vi "Reveal World.vi"(6 "radius":i32 min=0, 8 "y":i32 min=0, 9 "x":i32 min=0, 10 "cost in":dbl[][](array[numeric]), 11 "map reference in":refnum<data-value>) -> (2 "cost out":dbl[][](array[numeric]), 3 "map reference in 2":refnum<data-value>)   [LabVIEW 2012]
uses:
  <vilib>/robotics/Navigation/shared/WorldMap/OccupancyGridWorldMap/NI_Robotics_OccupancyGridWorldMap.lvclass
panel:
  in  "error in (no error)":errorcluster
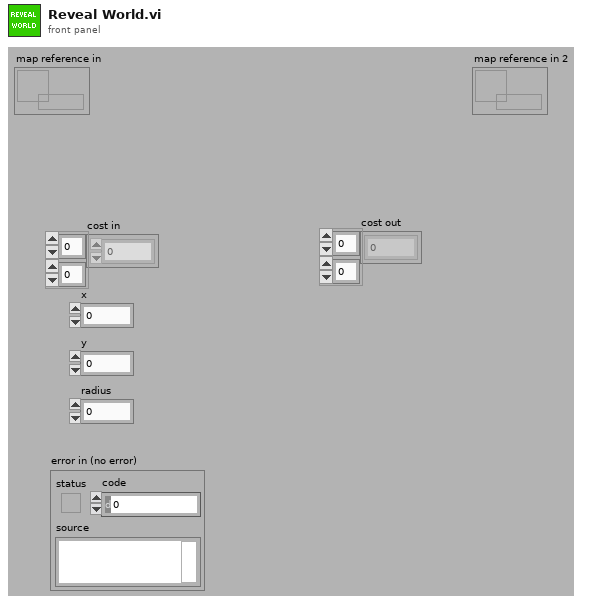
[diagram p1: front panel]
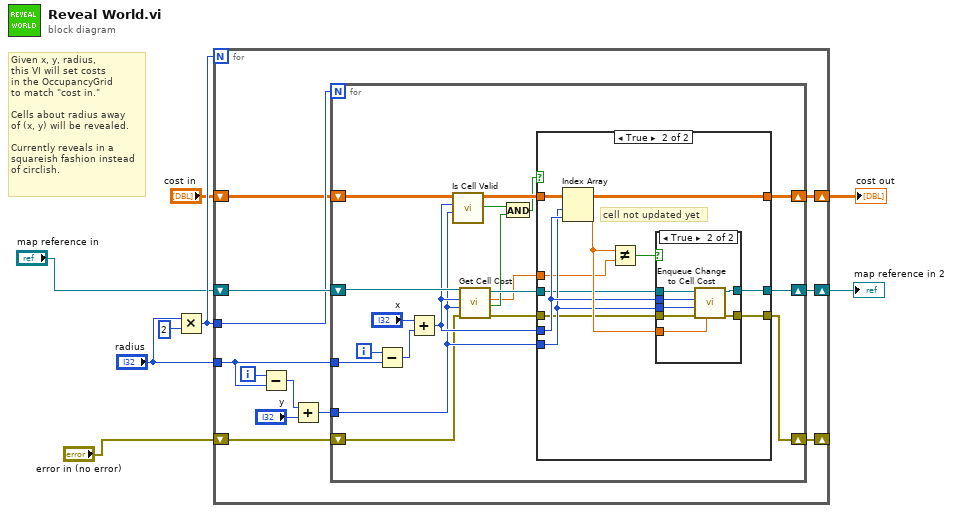
[diagram p0: block diagram]
diagram:
  # "Given x, y, radius,\nthis VI will set costs\nin the OccupancyGrid\nto match \"cost in.\"\n\nCells about radius away\nof (x, y) will be revealed.\n\nCurrently reveals in a \nsquareish fashion instead\nof circlish."
  n1 = Multiply(x="radius", y=2) -> (x*y=w6:i32)
  n2 = for {
    N: w6 -> [_]
    shift-right: [w19] -> w2
    shift-left: "map reference in" -> [w20]
    tunnel: w6 -> [w18]
    tunnel: "radius" -> [w16]
    shift-right: [w14] -> w4
    shift-left: "cost in" -> [w15]
    shift-right: [w9] -> _
    shift-left: "error in (no error)" -> [w10]
    i -> [w17]
    n3 = Subtract(x=w17, y=w16) -> (x-y=w13:i32)
    n4 = Add(x=w13, y="y") -> (x+y=w11:i32)
    n5 = for {
      N: w18 -> [_]
      shift-right: [w39] -> w19
      shift-left: w20 -> [w29]
      tunnel: w16 -> [w37]
      tunnel: w11 -> [w26]
      shift-right: [w34] -> w14
      shift-left: w15 -> [w36]
      shift-right: [w21] -> w9
      shift-left: w10 -> [w23]
      i -> [w38]
      n6 = Subtract(x=w38, y=w37) -> (x-y=w32:i32)
      n7 = Add(x="x", y=w32) -> (x+y=w27:i32)
      n8 = call "Is Cell Valid.vi"("y"=w26, "x"=w27, "cost in"=w36) -> ("Valid"=w30:bool, "cost out"=w35:dbl[][])  [unwired: 7 in]
      n9 = call <vilib>:"Get Cell Cost.vi"("error in (no error)"=w23, "y"=w26, "x"=w27, "map reference in"=w29) -> ("error out"=w22:errorcluster, "found?"=w25:bool, "cost"=w24:dbl, "map reference out"=w28:refnum<data-value>)  [unwired: 4 in]
      n10 = And(x=w30, y=w25) -> (x .and. y?=w33:bool)
      n11 = case shown="True" w33 {
        tunnel: [w42 w52] -> w39
        tunnel: w28 -> [w42 w46]
        tunnel: w27 -> [_ w49]
        tunnel: w26 -> [_ w48]
        tunnel: w35 -> [w41 w43]
        tunnel: [w41 w43] -> w34
        tunnel: w24 -> [_ w47]
        tunnel: w22 -> [w40 w45]
        tunnel: [w40 w44] -> w21
        frame False {
        }
        frame True {
          # "cell not updated yet"
          n12 = Index Array(array=w43, index (row)=w48, index (col)=w49) -> (element=w50:dbl)
          n13 = Not Equal?(x=w50, y=w47) -> (x != y?=w51:bool)
          n14 = case shown="True" w51 {
            tunnel: [w54 w57] -> w52
            tunnel: w46 -> [w54 w61]
            tunnel: w49 -> [_ w60]
            tunnel: w48 -> [_ w59]
            tunnel: w50 -> [_ w58]
            tunnel: w45 -> [w53 w56]
            tunnel: [w53 w55] -> w44
            frame False {
            }
            frame True {
              n15 = call <vilib>:"Enqueue Change to Cell Cost.vi"("cost"=w58, "error in (no error)"=w56, "y"=w59, "x"=w60, "map reference in"=w61) -> ("error out"=w55:errorcluster, "map reference out"=w57:refnum<data-value>)  [unwired: 5 in]
            }
          }
        }
      }
    }
  }
  "cost out" <- w4
  "map reference in 2" <- w2
